vi "ukol3.vi"() -> ()   [LabVIEW 2023]
uses:
  <vilib>/Analysis/4window.llb/windowTd.ctl
  <vilib>/Analysis/baseanly.llb/Mean (DBL).vi
  <vilib>/measure/maspectr.llb/FFT Spectrum (Mag-Phase) for 1 Chan.vi
  <vilib>/measure/NI_MABase.lvlib
  <vilib>/measure/NI_MAPro.lvlib
  <vilib>/Analysis/NI_AALPro.lvlib
  <vilib>/Analysis/NI_AALBase.lvlib
panel:
  out "Waveform Graph":cluster{"f0":dbl, "df":dbl, "magnitude":dbl[]}(graph)
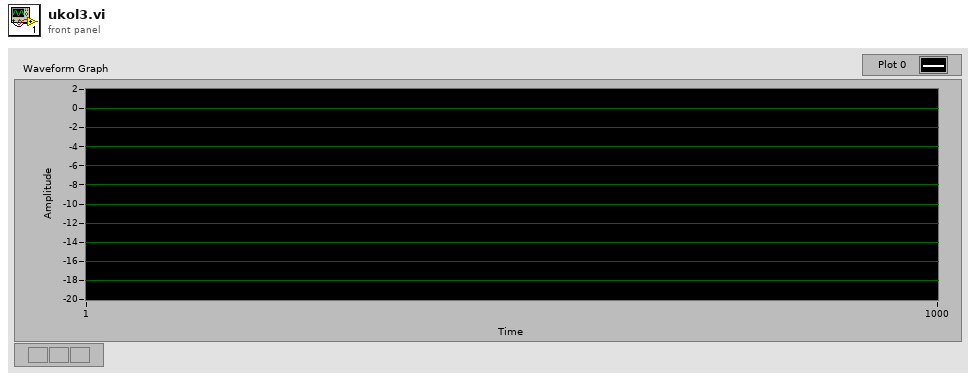
[diagram p1: front panel]
types:
  T1 = cluster{"dB On (F)":bool, "unwrap phase (F)":bool, "convert to degree (F)":bool}
  T2 = typedef "NI_AALPro.lvlib/windowTd.ctl" = u32
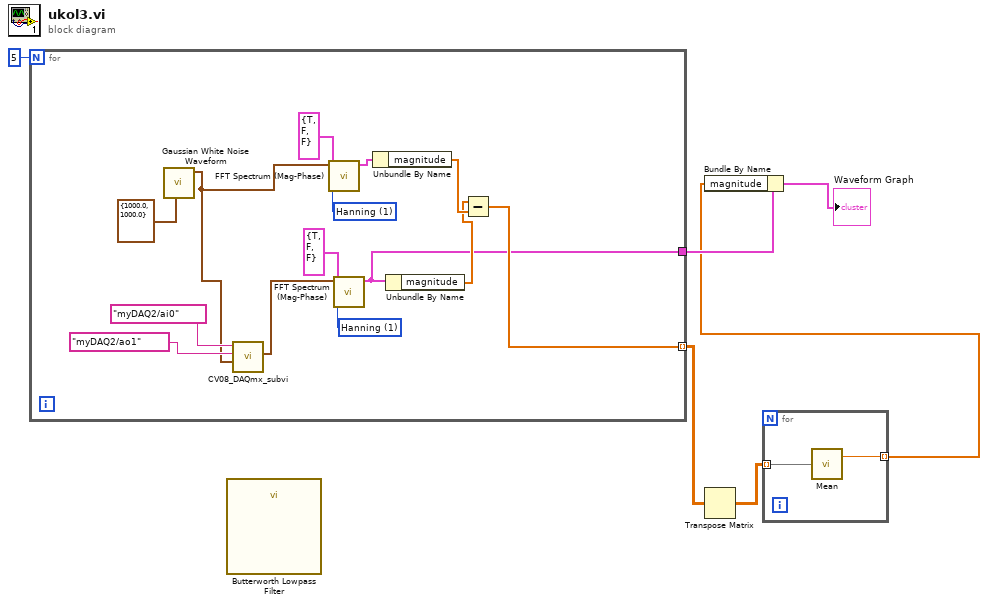
[diagram p0: block diagram]
diagram:
  n1 = for {
    N: 5 -> [_]
    tunnel: [w8] -> w2 mode=indexing
    tunnel: [w7] -> w5
    w16 = T2 1 items=["Rectangle"=0, "Hanning"=1, "Hamming"=2, "Blackman-Harris"=3, "Exact Blackman"=4, "Blackman"=5, "Flat Top"=6, "4 Term B-Harris "=7, "7 Term B-Harris"=8, "Low Sidelobe"=9, "Blackman Nuttall"=11, "Triangle"=30, "Bartlett-Hanning"=31, "Bohman"=32, "Parzen"=33, "Welch"=34, "Kaiser"=60, "Dolph-Chebyshev"=61, "Gaussian"=62] ("window")
    w18 = T2 1 items=["Rectangle"=0, "Hanning"=1, "Hamming"=2, "Blackman-Harris"=3, "Exact Blackman"=4, "Blackman"=5, "Flat Top"=6, "4 Term B-Harris "=7, "7 Term B-Harris"=8, "Low Sidelobe"=9, "Blackman Nuttall"=11, "Triangle"=30, "Bartlett-Hanning"=31, "Bohman"=32, "Parzen"=33, "Welch"=34, "Kaiser"=60, "Dolph-Chebyshev"=61, "Gaussian"=62] ("window")
    n2 = call <vilib>:"Gaussian White Noise Waveform.vi"("sampling info"=cluster{"Fs":dbl, "#s":dbl} {"Fs"=1000.0, "#s"=1000.0}) -> ("signal out"=w12:waveform(dbl))  [unwired: 9 in, 1 out]
    n3 = call "CV08_DAQmx_subvi.vi"("data in"=w12, "AO channel"=tag "myDAQ2/ao1", "AI channel"=tag "myDAQ2/ai0") -> ("data out"=w13:waveform(dbl))  [unwired: 7 in, 1 out]
    n4 = call-poly <vilib>:"FFT Spectrum (Mag-Phase).vi"("view"=T1 {"dB On (F)"=TRUE, "unwrap phase (F)"=FALSE, "convert to degree (F)"=FALSE}, "window"=w16, "time signal"=w12) -> ("magnitude"=w11:cluster{"f0":dbl, "df":dbl, "magnitude":dbl[]})  [unwired: 4 in, 4 out]
    n5 = call-poly <vilib>:"FFT Spectrum (Mag-Phase).vi"("view"=T1 {"dB On (F)"=TRUE, "unwrap phase (F)"=FALSE, "convert to degree (F)"=FALSE}, "window"=w18, "time signal"=w13) -> ("magnitude"=w7:cluster{"f0":dbl, "df":dbl, "magnitude":dbl[]})  [unwired: 4 in, 4 out]
    n6 = Unbundle By Name(w11) -> ("magnitude"=w10:dbl[])
    n7 = Unbundle By Name(w7) -> ("magnitude"=w9:dbl[])
    n8 = Subtract(x=w9, y=w10) -> (x-y=w8:dbl[])
  }
  n9 = call "Butterworth Lowpass Filter"() -> ()  [unwired: 10 in, 2 out]
  n10 = Transpose Matrix(1:w2) -> (0:w1:dbl[][])
  n11 = for {
    tunnel: w1 -> [w22] mode=indexing
    tunnel: [w21] -> w3 mode=indexing
    n12 = call-poly <vilib>:"Mean.vi"("X"=w22) -> ("mean"=w21:dbl)  [unwired: 1 out]
  }
  n13 = Bundle By Name(cluster=w5, "magnitude"=w3) -> (→"Waveform Graph":cluster{"f0":dbl, "df":dbl, "magnitude":dbl[]})
